vi "ScreenGrabberMain.vi"(8 "Error In":errorcluster, 9 "Grabber Timer":dbl=5.0 min=0.0 max=60.0, 10 "Grab Window every":u32=10 min=10 max=2000 step=10, 11 "Window Title":string="Assetto Corsa") -> (0 "ErrorOut":errorcluster)   [LabVIEW 2018, in "ScreenGrabber.lvlib"]
uses:
  ScreenGrabber.lvlib
  Controls/PreferredControlMethod.ctl
  Controls/PreferredSavingConvention.ctl
  Controls/QueueDriverStates.ctl
  Controls/TemplateDataCluster.ctl
  <vilib>/picture/picture.llb/imagedata.ctl
  System.Drawing
  USER32.DLL
  <vilib>/wsapi/NI_WebServices.lvlib
panel:
  out "Slider":u32(slide) caption="Idle" scale=0.0..100.0
  out "TimerBeforeStart":string
  in  "NamingConvention":T1
  in  "About":bool
  in  "Movement Buttons":T2
  in  "Stop":bool
  in  "Start Grabber":bool
  # "SCREEN GRABBER"
  # "(Verbatim Window Title of  the screen to be grabbed)"
  # "(millisecs)"
  # "(Timer secs)"
  # "Preferred Control"
  # "Naming Convention"
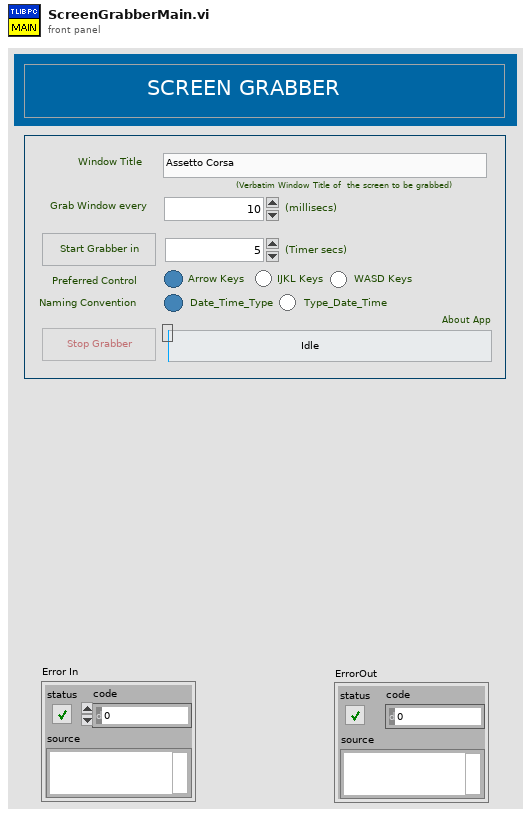
[diagram p1: front panel]
types:
  T1 = typedef "ScreenGrabber.lvlib/PreferredSavingConvention.ctl" = enum32{"Date_Time_Type", "Type_Date_Time"}
  T2 = typedef "ScreenGrabber.lvlib/PreferredControlMethod.ctl" = enum32{"Arrow Keys  ", "IJKL Keys", "WASD Keys"}
  T3 = typedef "ScreenGrabber.lvlib/TemplateDataCluster.ctl" = cluster{"UpVkeyCode":i16, "DownVkeyCode":i16, "LeftVkeyCode":i16, "RightVkeyCode":i16, "WindowHandle":u32, "WindowDimensions":i32[], "WindowWidth":i32, "WindowHeight":i32, "ImageType":u32, "MemoryStreamRef":refnum<k24>, "ImageRef":refnum<k24>, "GraphicsRef":refnum<k24>, "PNGformatRef":refnum<k24>, "ImageSizeRef":refnum<k24>, "CurrentImageData":T4, "SavingConvention":string, "Array of Images":cluster{"CurrentImageData":T4, "Image Path":path}[]}
  T4 = typedef "imagedata.ctl" = cluster{"image type":i32, "image depth":i32, "image":u8[], "mask":u8[], "colors":u32[], "Rectangle":cluster{"left":i16, "top":i16, "right":i16, "bottom":i16}}
  T5 = typedef "ScreenGrabber.lvlib/QueueDriverStates.ctl" = enum16{"Create", "Enqueue", "Enqueue N", "Dequeue", "Enstack", "Enstack N", "Flush", "Destroy"}
  T6 = enum8{"Enabled", "Disabled", "Disabled and Grayed Out"}
  T7 = cluster{"CurrentImageData":T4, "Image Path":path}
  T8 = cluster{"CurrentImageData":T4, "Image Path":path}[]
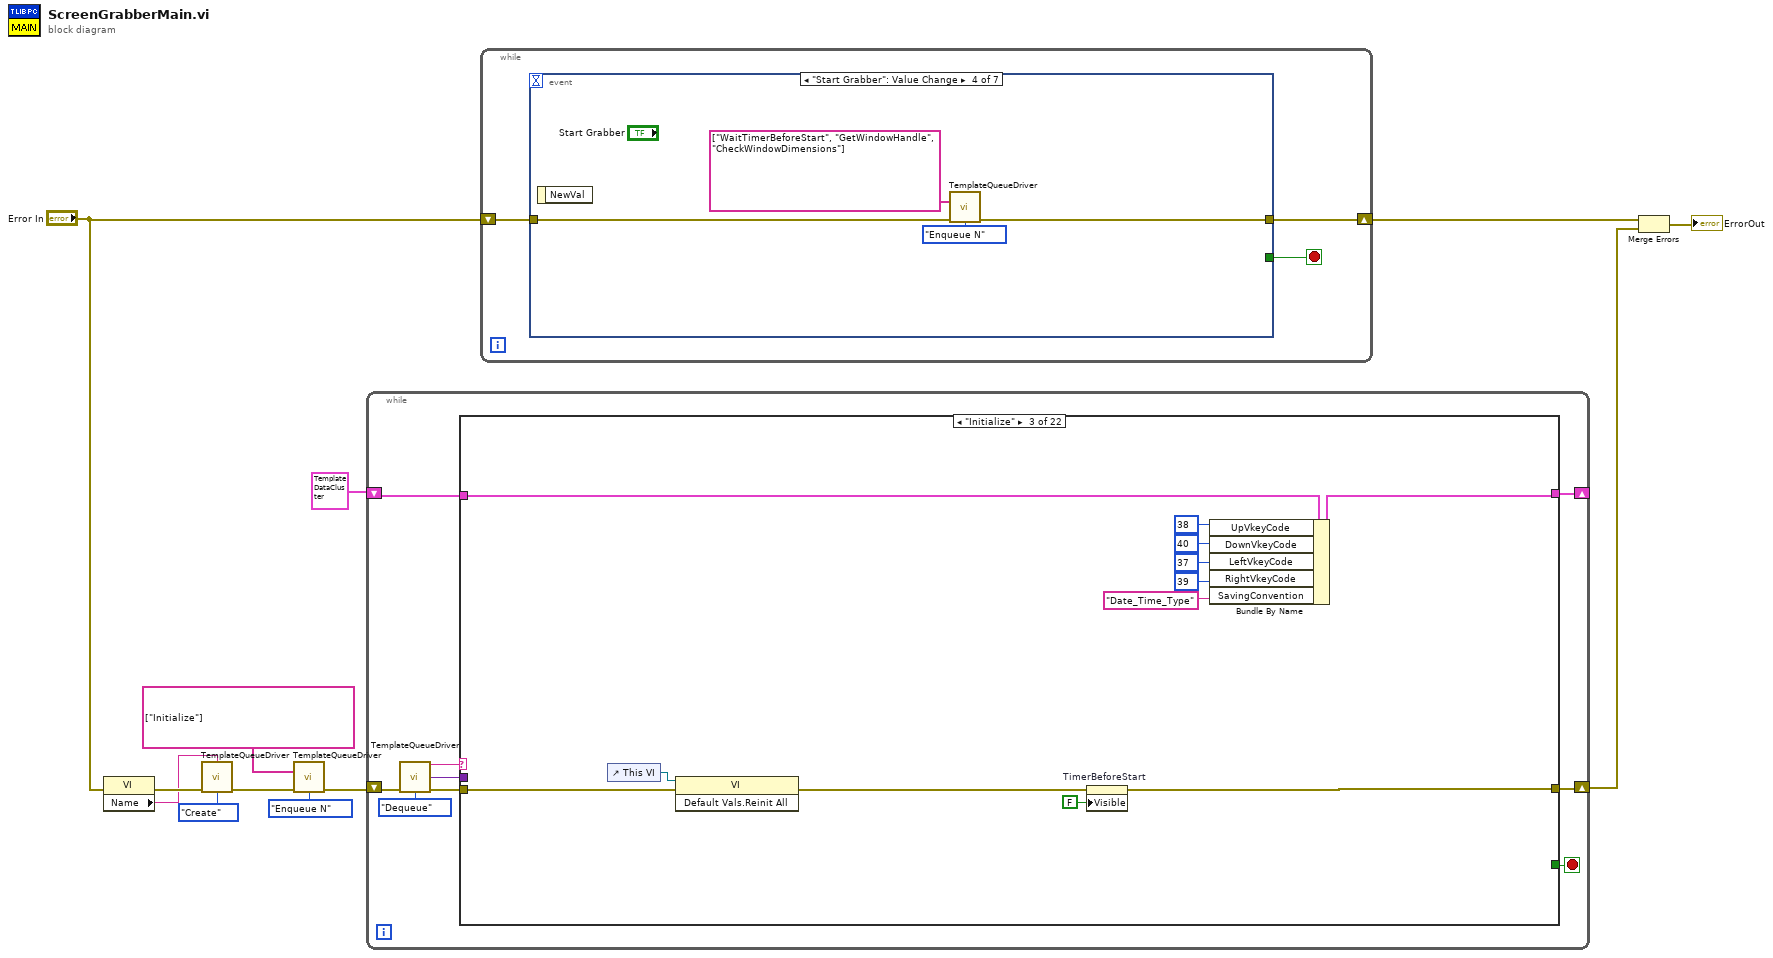
[diagram p0: block diagram]
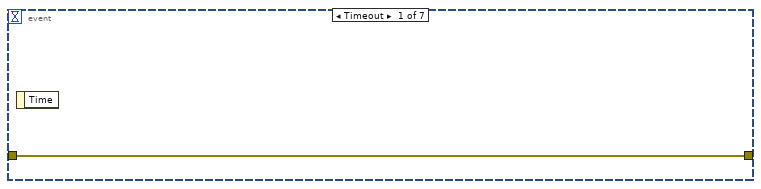
[diagram p2: hidden frame]
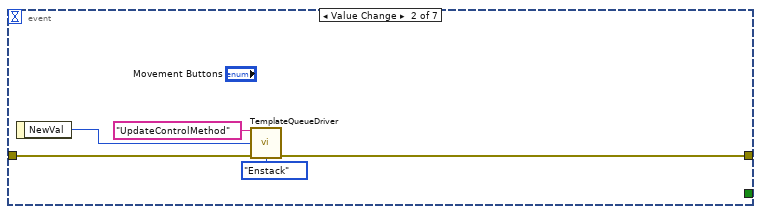
[diagram p3: hidden frame]
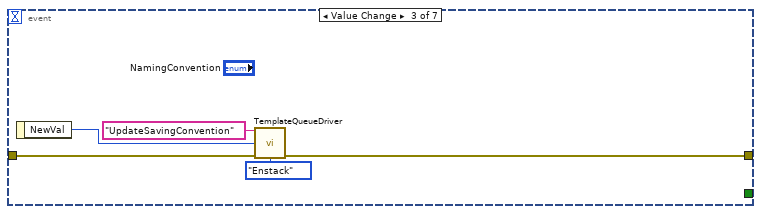
[diagram p4: hidden frame]
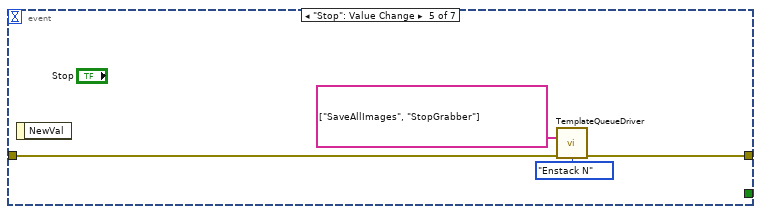
[diagram p5: hidden frame]
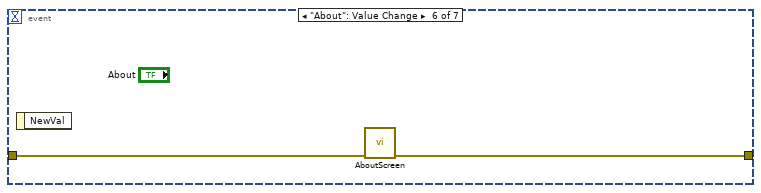
[diagram p6: hidden frame]
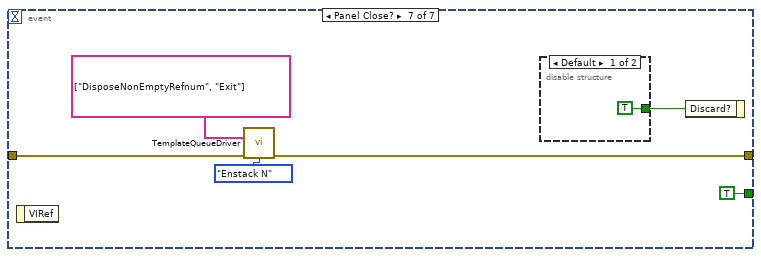
[diagram p7: hidden frame]
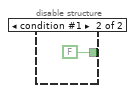
[diagram p8: hidden frame]
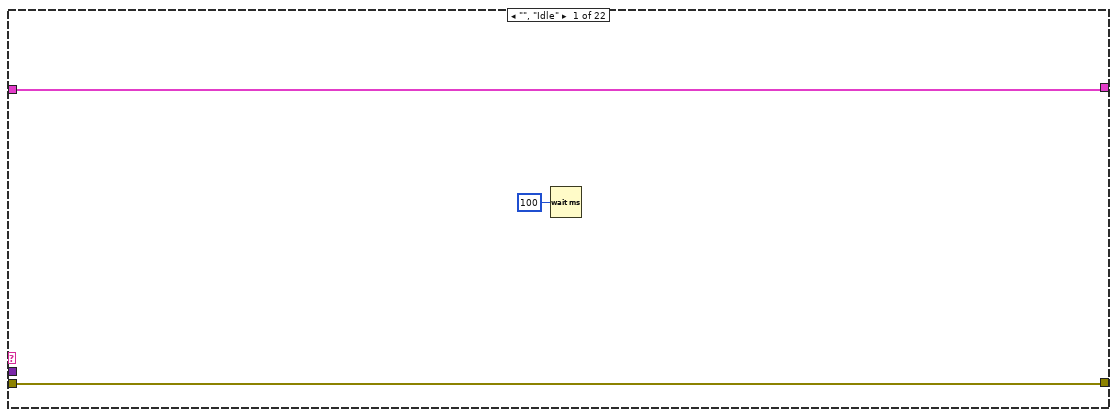
[diagram p9: hidden frame]
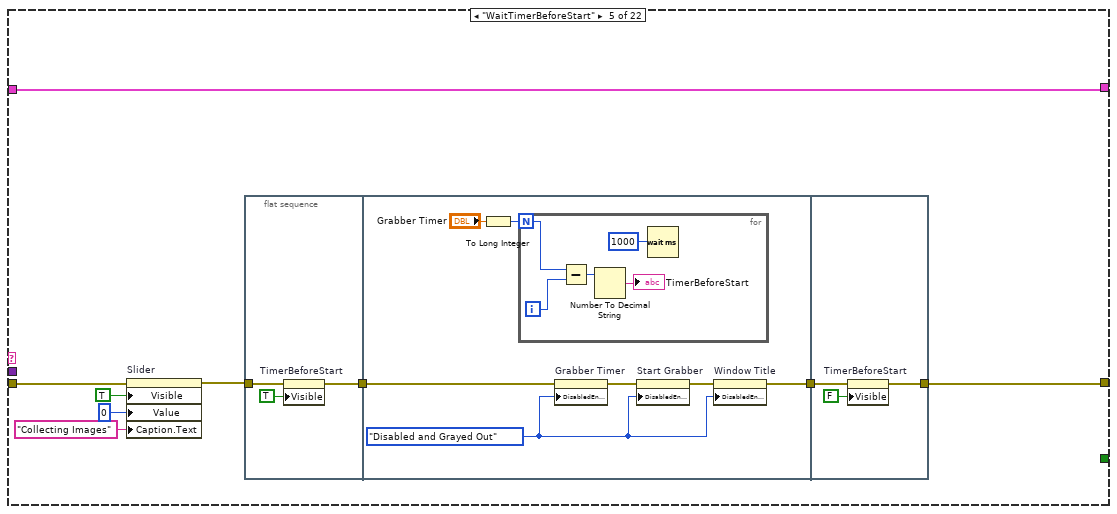
[diagram p12: hidden frame]
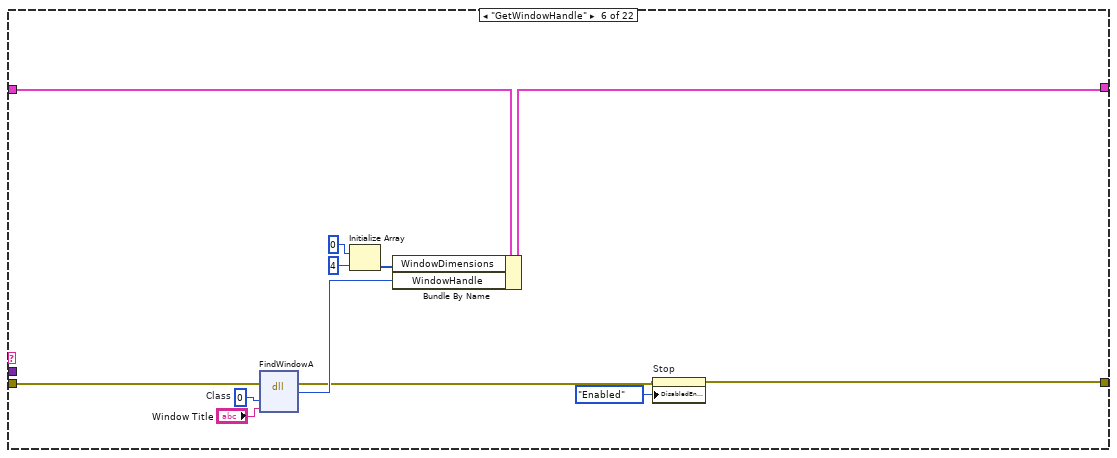
[diagram p13: hidden frame]
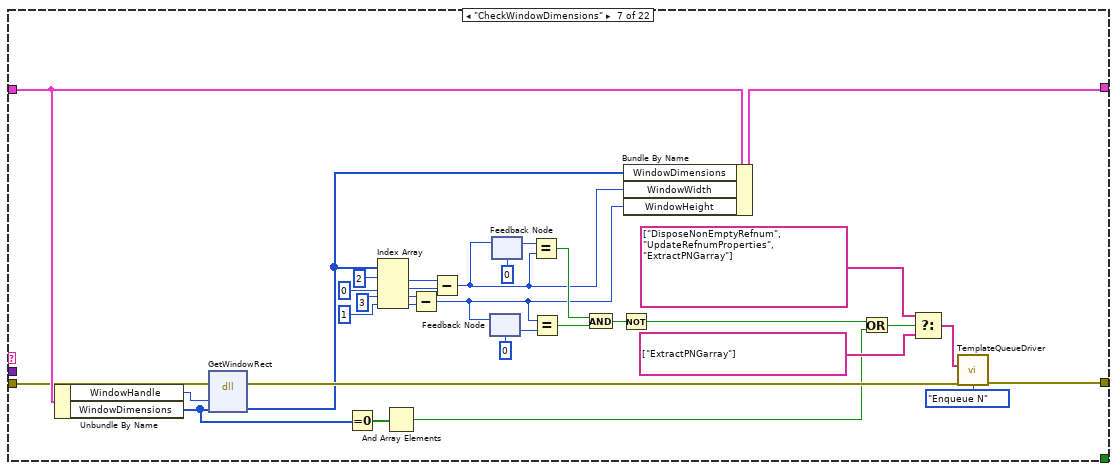
[diagram p14: hidden frame]
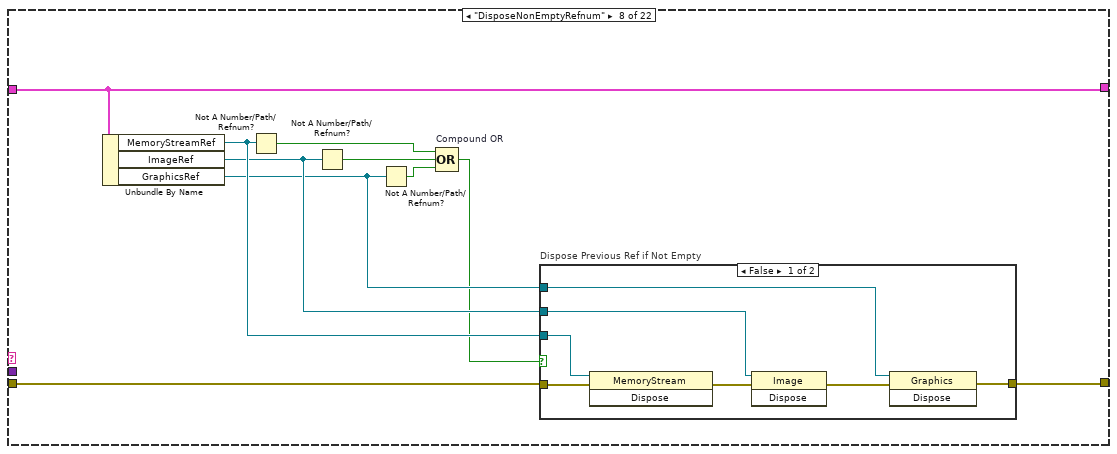
[diagram p15: hidden frame]
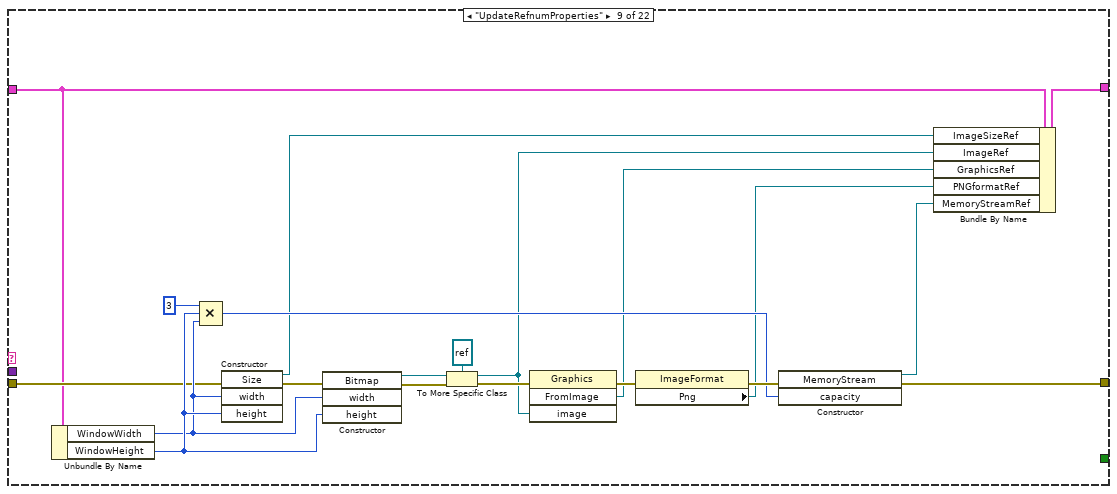
[diagram p17: hidden frame]
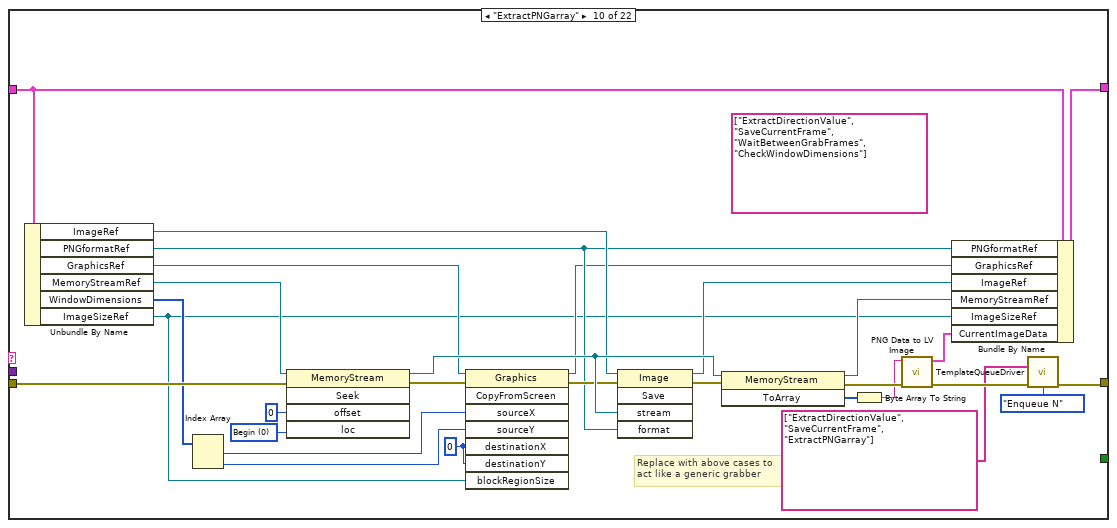
[diagram p18: hidden frame]
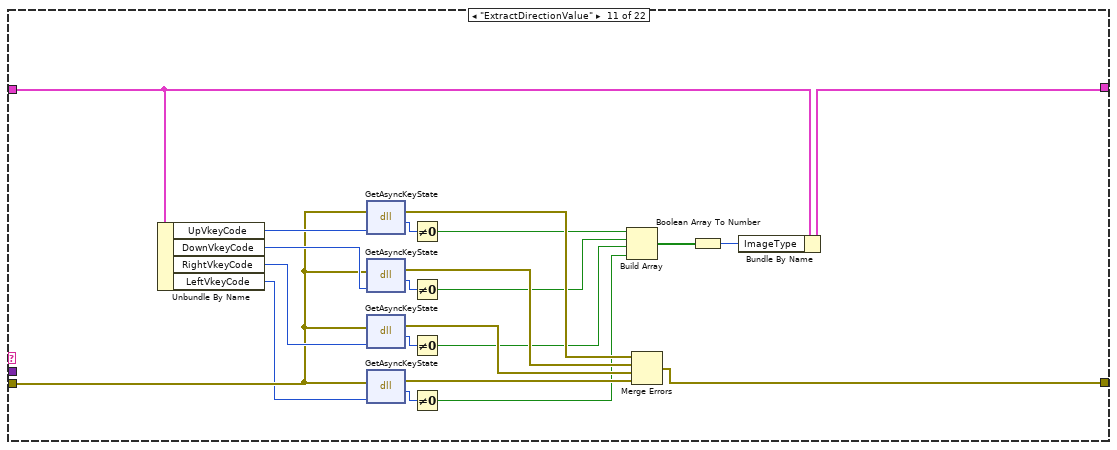
[diagram p19: hidden frame]
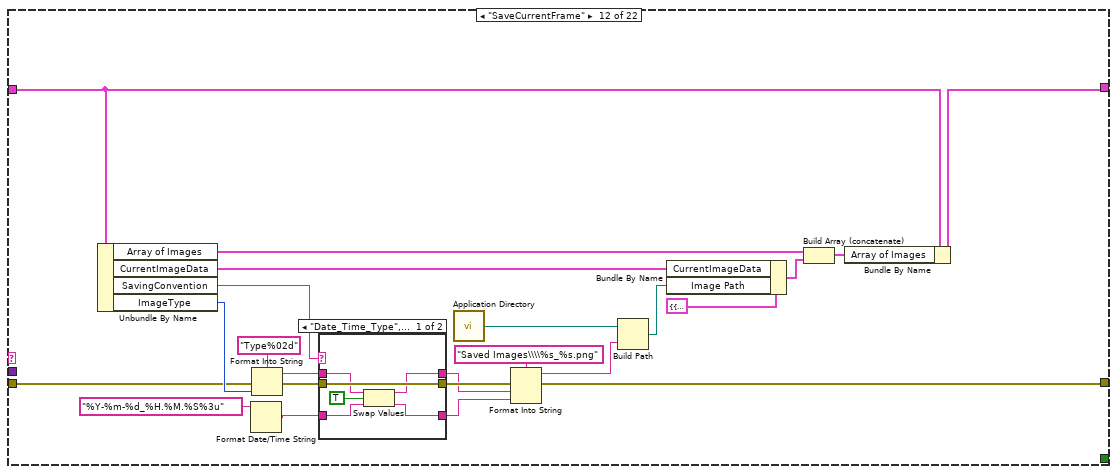
[diagram p20: hidden frame]
diagram:
  n1 = property class="VI"(error in="Error In") -> (error out=w6:errorcluster, "Name"=w5:string)  [unwired: 1 in, 1 out]
  n2 = call "TemplateQueueDriver.vi"("Name"=w5, "ErrorIn"=w6, "Operation"=QueueDriverStates."Create") -> ("ErrorOut"=w12:errorcluster)  [unwired: 10 in, 2 out]
  n3 = call "TemplateQueueDriver.vi"("States[]"=string[] ["Initialize"], "ErrorIn"=w12, "Operation"=QueueDriverStates."Enqueue N") -> ("ErrorOut"=w11:errorcluster)  [unwired: 10 in, 2 out]
  n4 = while {
    shift-right: [w18] -> w10
    shift-left: w11 -> [w21]
    shift-right: [w16] -> _
    shift-left: T3 {"UpVkeyCode"=0, "DownVkeyCode"=0, "LeftVkeyCode"=0, "RightVkeyCode"=0, "WindowHandle"=0, "WindowDimensions"=[], "WindowWidth"=0, "WindowHeight"=0, "ImageType"=0, "MemoryStreamRef"=refnum, "ImageRef"=refnum, "GraphicsRef"=refnum, "PNGformatRef"=refnum, "ImageSizeRef"=refnum, "CurrentImageData"={"image type"=0, "image depth"=0, "image"=[], "mask"=[], "colors"=[], "Rectangle"={"left"=0, "top"=0, "right"=0, "bottom"=0}}, "SavingConvention"="", "Array of Images"=[]} -> [w15]
    stop <- w17 stop-if-true
    n5 = call "TemplateQueueDriver.vi"("ErrorIn"=w21, "Operation"=QueueDriverStates."Dequeue") -> ("State"=w19:string, "Data"=w13:variant, "ErrorOut"=w20:errorcluster)  [unwired: 11 in]
    n6 = case shown="\"Initialize\"" w19 {
      selector: w19 -> [_ _ _ _ _ _ _ _ _ _ _ _ _ _ _ _ _ _ _ _ _ w358]
      tunnel: w20 -> [w24 w26 w36 w40 w45 w79 w110 w121 w138 w171 w189 w204 w236 w249 w285 w299 w310 w331 w333 w336 w342 w357]
      tunnel: [w24 w26 w27 w40 w48 w69 w91 w113 w141 w152 w196 w202 w236 w247 w284 w299 w309 w323 w333 w334 w351 w356] -> w18
      tunnel: [_ _ _ _ _ _ _ _ _ _ _ _ _ _ _ _ _ _ _ _ TRUE _] -> w17
      tunnel: w15 -> [w23 w25 w38 w39 w49 w71 w111 w122 w136 w156 w180 w222 w235 w253 w286 w298 w300 w328 w332 w337 w349 w355]
      tunnel: [w23 w25 w37 w39 w49 w72 w112 w122 w137 w157 w181 w211 w235 w253 w277 w298 w301 w329 w332 w337 w349 w355] -> w16
      tunnel: w13 -> [_ _ _ _ _ _ _ _ _ _ _ _ _ _ _ _ w308 w330 _ _ _ _]
      frame "", "Idle" {
        n7 = Wait (ms)(milliseconds to wait=u32 100) -> ()  [unwired: 1 out]
      }
      frame "---------Initialization---------" {
      }
      frame "Initialize" {
        n8 = control-ref of="This VI"() -> (w35:refnum<vi>)
        n9 = invoke class="VI" method="Default Vals.Reinit All"(reference=w35, error in=w36) -> (error out=w28:errorcluster)  [unwired: 1 in, 2 out]
        n10 = property on="TimerBeforeStart" class="Str"(error in=w28, "Visible"=FALSE) -> (error out=w27:errorcluster)  [unwired: 1 in, 1 out]
        n11 = Bundle By Name(cluster=w38, "UpVkeyCode"=i16 38 ("nvirtkey"), "DownVkeyCode"=i16 40 ("nvirtkey"), "LeftVkeyCode"=i16 37 ("nvirtkey"), "RightVkeyCode"=i16 39 ("nvirtkey"), "SavingConvention"="Date_Time_Type" ("format string")) -> (w37:T3)
      }
      frame "-----------Functions----------" {
      }
      frame "WaitTimerBeforeStart" {
        n12 = property on="Slider" class="Slide (strict)"(error in=w45, "Visible"=TRUE, "Value"=u32 0 ("Slider"), "Caption.Text"="Collecting Images") -> (error out=w44:errorcluster)  [unwired: 1 in, 1 out]
        n13 = flat-sequence {
          tunnel: w44 -> [w51]
          tunnel: [w50] -> w46
          tunnel: [w56] -> w47
          tunnel: w46 -> [w59]
          tunnel: [w65] -> w48
          tunnel: w47 -> [w66]
          frame #0 {
            n14 = property on="TimerBeforeStart" class="Str"(error in=w51, "Visible"=TRUE) -> (error out=w50:errorcluster)  [unwired: 1 in, 1 out]
          }
          frame #1 {
            w55 = T6."Disabled and Grayed Out" ("Disabled")
            n15 = To Long Integer(number="Grabber Timer") -> (32bit integer=w53:i32)
            n16 = for {
              N: w53 -> [w63]
              i -> [w62]
              n17 = Subtract(x=w63, y=w62) -> (x-y=w61:i32)
              n18 = Number To Decimal String(number=w61) -> (decimal integer string=→"TimerBeforeStart":string)  [unwired: 1 in]
              n19 = Wait (ms)(milliseconds to wait=u32 1000 ("y")) -> ()  [unwired: 1 out]
            }
            n20 = property on="Grabber Timer" class="DigNum (strict)"(error in=w59, "DisabledEnum"=w55) -> (error out=w58:errorcluster)  [unwired: 1 in, 1 out]
            n21 = property on="Start Grabber" class="Bool"(error in=w58, "DisabledEnum"=w55) -> (error out=w57:errorcluster)  [unwired: 1 in, 1 out]
            n22 = property on="Window Title" class="Str"(error in=w57, "DisabledEnum"=w55) -> (error out=w56:errorcluster)  [unwired: 1 in, 1 out]
          }
          frame #2 {
            n23 = property on="TimerBeforeStart" class="Str"(error in=w66, "Visible"=FALSE) -> (error out=w65:errorcluster)  [unwired: 1 in, 1 out]
          }
        }
      }
      frame "GetWindowHandle" {
        w77 = 0  # Class
        n24 = dll-call lib="USER32.DLL" fn="FindWindowA"(error in=w79, "class"=w77, "title"="Window Title") -> (error out=w70:errorcluster, "Window Handle"=w76:u32)  [unwired: 4 in, 1 out]
        n25 = Initialize Array(0, 4) -> (w73:i32[])
        n26 = Bundle By Name(cluster=w71, "WindowDimensions"=w73, "WindowHandle"=w76) -> (w72:T3)
        n27 = property on="Stop" class="Bool"(error in=w70, "DisabledEnum"=T6."Enabled" ("Disabled")) -> (error out=w69:errorcluster)  [unwired: 1 in, 1 out]
      }
      frame "CheckWindowDimensions" {
        n28 = Unbundle By Name(w111) -> ("WindowHandle"=w93:u32, "WindowDimensions"=w80:i32[])
        n29 = dll-call lib="USER32.DLL" fn="GetWindowRect"(error in=w110, "hWnd"=w93, "RECT"=w80) -> (error out=w92:errorcluster, "RECT"=w84:i32[])  [unwired: 4 in, 1 out]
        n30 = Equal To 0?(x=w80) -> (x = 0?=w85:bool[])
        n31 = Index Array(array=w84, index #1=2 ("index"), index #2=0 ("index"), index #3=3 ("index"), index #4=1 ("index")) -> (element #1=w105:i32, element #2=w104:i32, element #3=w103:i32, element #4=w102:i32)
        n32 = And Array Elements(Boolean array=w85) -> (logical AND=w81:bool)
        n33 = Subtract(x=w103, y=w102) -> (x-y=w94:i32)
        n34 = Subtract(x=w105, y=w104) -> (x-y=w95:i32)
        n35 = feedback #1(0) -> (w100:i32)
        n36 = feedback-in #1(w94) -> ()
        n37 = feedback #2(0) -> (w101:i32)
        n38 = feedback-in #2(w95) -> ()
        n39 = Equal?(x=w101, y=w95) -> (x = y?=w99:bool)
        n40 = Equal?(x=w94, y=w100) -> (x = y?=w98:bool)
        n41 = And(x=w99, y=w98) -> (x .and. y?=w89:bool)
        n42 = Not(x=w89) -> (.not. x?=w83:bool)
        n43 = Bundle By Name(cluster=w111, "WindowDimensions"=w84, "WindowWidth"=w95, "WindowHeight"=w94) -> (w112:T3)
        n44 = Or(x=w83, y=w81) -> (x .or. y?=w82:bool)
        n45 = Select(t=string[] ["DisposeNonEmptyRefnum", "UpdateRefnumProperties", "ExtractPNGarray"] ("States[]"), s=w82, f=string[] ["ExtractPNGarray"] ("States[]")) -> (s? t:f=w86:string[])
        n46 = call "TemplateQueueDriver.vi"("States[]"=w86, "ErrorIn"=w92, "Operation"=QueueDriverStates."Enqueue N") -> ("ErrorOut"=w91:errorcluster)  [unwired: 10 in, 2 out]
      }
      frame "DisposeNonEmptyRefnum" {
        n47 = Unbundle By Name(w122) -> ("MemoryStreamRef"=w120:refnum<k24>, "ImageRef"=w119:refnum<k24>, "GraphicsRef"=w118:refnum<k24>)
        n48 = Not A Number/Path/Refnum?(number/path/refnum=w120) -> (NaN/Path/Refnum?=w117:bool)
        n49 = Not A Number/Path/Refnum?(number/path/refnum=w119) -> (NaN/Path/Refnum?=w116:bool)
        n50 = Not A Number/Path/Refnum?(number/path/refnum=w118) -> (NaN/Path/Refnum?=w115:bool)
        n51 = Compound Arithmetic op=OR "Compound OR"(w117, w116, w115) -> (w114:bool)
        n52 = case "Dispose Previous Ref if Not Empty" shown="False" w114 {
          tunnel: [w127 w130] -> w113
          tunnel: w121 -> [w126 w130]
          tunnel: w120 -> [w125 _]
          tunnel: w119 -> [w124 _]
          tunnel: w118 -> [w123 _]
          frame False {
            n53 = invoke class="MemoryStream" method="Dispose"(reference=w125, error in=w126) -> (error out=w128:errorcluster)  [unwired: 1 in, 2 out]
            n54 = invoke class="Image" method="Dispose"(reference=w124, error in=w128) -> (error out=w129:errorcluster)  [unwired: 1 in, 2 out]
            n55 = invoke class="Graphics" method="Dispose"(reference=w123, error in=w129) -> (error out=w127:errorcluster)  [unwired: 1 in, 2 out]
          }
          frame True {
          }
        }
      }
      frame "UpdateRefnumProperties" {
        n56 = Unbundle By Name(w136) -> ("WindowWidth"=w139:i32, "WindowHeight"=w144:i32)
        n57 = Compound Arithmetic op=MULTIPLY(3 ("value"), w144, w139) -> (w140:i32)
        n58 = constructor class="Size"(error in=w138, "width"=w139, "height"=w144) -> (reference out=w131:refnum<k24>, error out=w145:errorcluster)  [unwired: 2 in, 3 out]
        n59 = constructor class="Bitmap"(error in=w145, "width"=w139, "height"=w144) -> (reference out=w150:refnum<k24>, error out=w148:errorcluster)  [unwired: 2 in, 3 out]
        n60 = To More Specific Class(target class=refnum<k24> refnum, reference=w150, error in=w148) -> (specific class reference=w132:refnum<k24>, error out=w147:errorcluster)
        n61 = invoke class="Graphics" method="FromImage"(error in=w147, "image"=w132) -> (error out=w146:errorcluster, "FromImage"=w133:refnum<k24>)  [unwired: 2 in, 2 out]
        n62 = property class="ImageFormat"(error in=w146) -> (error out=w142:errorcluster, "Png"=w134:refnum<k24>)  [unwired: 1 in, 1 out]
        n63 = constructor class="MemoryStream"(error in=w142, "capacity"=w140) -> (reference out=w135:refnum<k24>, error out=w141:errorcluster)  [unwired: 2 in, 2 out]
        n64 = Bundle By Name(cluster=w136, "ImageSizeRef"=w131, "ImageRef"=w132, "GraphicsRef"=w133, "PNGformatRef"=w134, "MemoryStreamRef"=w135) -> (w137:T3)
      }
      frame "ExtractPNGarray" {
        (unwired) string[] ["ExtractDirectionValue", "SaveCurrentFrame", "WaitBetweenGrabFrames", "CheckWindowDimensions"] ("States[]")
        w174 = 0 ("destinationX")
        w178 = 0 items=["Begin", "Current", "End"] ("loc")
        # "Replace with above cases to \nact like a generic grabber"
        n65 = Unbundle By Name(w156) -> ("ImageRef"=w165:refnum<k24>, "PNGformatRef"=w163:refnum<k24>, "GraphicsRef"=w166:refnum<k24>, "MemoryStreamRef"=w170:refnum<k24>, "WindowDimensions"=w169:i32[], "ImageSizeRef"=w160:refnum<k24>)
        n66 = Index Array(array=w169) -> (element #1=w167:i32, element #2=w168:i32)  [unwired: 2 in]
        n67 = invoke class="MemoryStream" method="Seek"(reference=w170, error in=w171, "offset"=i64 0, "loc"=w178) -> (reference out=w177:refnum<k24>, error out=w176:errorcluster)  [unwired: 1 in, 3 out]
        n68 = invoke class="Graphics" method="CopyFromScreen"(reference=w166, error in=w176, "sourceX"=w167, "sourceY"=w168, "destinationX"=w174, "destinationY"=w174, "blockRegionSize"=w160) -> (reference out=w161:refnum<k24>, error out=w175:errorcluster)  [unwired: 1 in, 6 out]
        n69 = invoke class="Image" method="Save"(reference=w165, error in=w175, "stream"=w177, "format"=w163) -> (reference out=w162:refnum<k24>, error out=w173:errorcluster)  [unwired: 1 in, 3 out]
        n70 = invoke class="MemoryStream" method="ToArray"(reference=w177, error in=w173) -> (reference out=w164:refnum<k24>, error out=w159:errorcluster, "ToArray"=w172:u8[])  [unwired: 1 in]
        n71 = Byte Array To String(unsigned byte array=w172) -> (string=w158:string)
        n72 = call <vilib>:"PNG Data to LV Image.vi"("error in (no error)"=w159, "png data"=w158) -> ("error out"=w153:errorcluster, "image data"=w155:T4)  [unwired: 8 in]
        n73 = Bundle By Name(cluster=w156, "PNGformatRef"=w163, "GraphicsRef"=w161, "ImageRef"=w162, "MemoryStreamRef"=w164, "ImageSizeRef"=w160, "CurrentImageData"=w155) -> (w157:T3)
        n74 = call "TemplateQueueDriver.vi"("States[]"=string[] ["ExtractDirectionValue", "SaveCurrentFrame", "ExtractPNGarray"], "ErrorIn"=w153, "Operation"=QueueDriverStates."Enqueue N") -> ("ErrorOut"=w152:errorcluster)  [unwired: 10 in, 2 out]
      }
      frame "ExtractDirectionValue" {
        n75 = Unbundle By Name(w180) -> ("UpVkeyCode"=w192:i16, "DownVkeyCode"=w191:i16, "RightVkeyCode"=w190:i16, "LeftVkeyCode"=w188:i16)
        n76 = dll-call lib="user32.dll" fn="GetAsyncKeyState"(error in=w189, "vKey"=w192) -> (error out=w195:errorcluster, "return type"=w198:u16)  [unwired: 3 in, 1 out]
        n77 = dll-call lib="user32.dll" fn="GetAsyncKeyState"(error in=w189, "vKey"=w191) -> (error out=w194:errorcluster, "return type"=w199:u16)  [unwired: 3 in, 1 out]
        n78 = dll-call lib="user32.dll" fn="GetAsyncKeyState"(error in=w189, "vKey"=w190) -> (error out=w193:errorcluster, "return type"=w200:u16)  [unwired: 3 in, 1 out]
        n79 = dll-call lib="user32.dll" fn="GetAsyncKeyState"(error in=w189, "vKey"=w188) -> (error out=w197:errorcluster, "return type"=w201:u16)  [unwired: 3 in, 1 out]
        n80 = Not Equal To 0?(x=w198) -> (x != 0?=w187:bool)
        n81 = Not Equal To 0?(x=w199) -> (x != 0?=w186:bool)
        n82 = Not Equal To 0?(x=w200) -> (x != 0?=w185:bool)
        n83 = Not Equal To 0?(x=w201) -> (x != 0?=w184:bool)
        n84 = Build Array(w187, w186, w185, w184) -> (w183:bool[])
        n85 = Merge Errors(w195, w194, w193, w197) -> (w196:errorcluster)
        n86 = Boolean Array To Number(Boolean array=w183) -> (number=w182:u32)
        n87 = Bundle By Name(cluster=w180, "ImageType"=w182) -> (w181:T3)
      }
      frame "SaveCurrentFrame" {
        n88 = Unbundle By Name(w222) -> ("Array of Images"=w209:T8, "CurrentImageData"=w206:T4, "SavingConvention"=w218:string, "ImageType"=w220:u32)
        n89 = Format Date/Time String(time format string (%c)="%Y-%m-%d_%H.%M.%S%3u") -> (date/time string=w212:string)  [unwired: 2 in]
        n90 = Format Into String(format string="Type%02d", error in=w204, w220) -> (resulting string=w215:string, error out=w217:errorcluster)  [unwired: 1 in]
        n91 = case shown="\"Date_Time_Type\", Default" w218 {
          tunnel: w217 -> [w230 w233]
          tunnel: [w230 w233] -> w216
          tunnel: w215 -> [w229 w232]
          tunnel: w212 -> [w227 w231]
          tunnel: [w228 w232] -> w214
          tunnel: [w226 w231] -> w213
          frame "Date_Time_Type", Default {
            n92 = Swap Values(12:w229, 13:TRUE ("?(T)"), 14:w227) -> (1:w228:string, 3:w226:string)
          }
          frame "Type_Date_Time" {
          }
        }
        n93 = call <vilib>:"Application Directory.vi"() -> ("Application Directory"=w203:path)
        n94 = Format Into String(format string="Saved Images\\\\%s_%s.png", error in=w216, w214, w213) -> (resulting string=w223:string, error out=w202:errorcluster)  [unwired: 1 in]
        n95 = Build Path(base path=w203, name or relative path=w223) -> (appended path=w205:path)
        n96 = Bundle By Name(cluster=T7 {"CurrentImageData"={"image type"=0, "image depth"=0, "image"=[], "mask"=[], "colors"=[], "Rectangle"={"left"=0, "top"=0, "right"=0, "bottom"=0}}, "Image Path"=path ""} ("Cluster"), "CurrentImageData"=w206, "Image Path"=w205) -> (w207:T7)
        n97 = Build Array (concatenate)(w209, w207) -> (w208:T8)
        n98 = Bundle By Name(cluster=w222, "Array of Images"=w208) -> (w211:T3)
      }
      frame "WaitBetweenGrabFrames" {
        n99 = Wait (ms)(milliseconds to wait="Grab Window every") -> ()  [unwired: 1 out]
      }
      frame "SaveAllImages" {
        n100 = call <vilib>:"Set Busy.vi"("error in (no error)"=w249) -> ("error out"=w241:errorcluster)  [unwired: 9 in, 1 out]
        n101 = call <vilib>:"Application Directory.vi"() -> ("Application Directory"=w243:path)
        n102 = Build Path(base path=w243, name or relative path="Saved Images" ("string")) -> (appended path=w244:path)
        n103 = call <vilib>:"Check if File or Folder Exists.vi"("error in (no error)"=w241, "path"=w244) -> ("error out"=w240:errorcluster, "file or folder exists?"=w239:bool, "dup path"=w238:path)  [unwired: 7 in]
        n104 = case "Create Folder\nif necessary" shown="False" w239 {
          tunnel: w240 -> [w256 w257]
          tunnel: [w255 w257] -> w237
          tunnel: w238 -> [w254 _]
          frame False {
            n105 = Create Folder(path (use dialog)=w254, error in=w256) -> (error out=w255:errorcluster)  [unwired: 1 in, 2 out]
          }
          frame True {
          }
        }
        n106 = property on="Stop" class="Bool"(error in=w237, "DisabledEnum"=T6."Disabled and Grayed Out" ("Disabled")) -> (error out=w246:errorcluster)  [unwired: 1 in, 1 out]
        n107 = Unbundle By Name(w253) -> ("Array of Images"=w252:T8)
        n108 = property on="Slider" class="Slide (strict)"(error in=w246, "Visible"=TRUE) -> (error out=w250:errorcluster)  [unwired: 1 in, 1 out]
        n109 = for {
          N -> [w265]
          tunnel: w252 -> [w272] mode=indexing
          tunnel: w250 -> [w273]
          tunnel: [w260] -> w248
          i -> [w266]
          w274 = 1  # Compression
          n110 = Unbundle By Name(w272) -> ("Image Path"=w270:path, "CurrentImageData"=w271:T4)
          n111 = Increment(x=w266) -> (x+1=w264:i32)
          n112 = Divide(x=w264, y=w265) -> (x/y=w269:dbl)
          n113 = Multiply(x=w269, y=100.0) -> (x*y=w267:dbl)
          n114 = call <vilib>:"Write PNG File.vi"("compression (default)"=w274, "error in (no error)"=w273, "image data"=w271, "path to PNG file"=w270) -> ("error out"=w261:errorcluster)  [unwired: 6 in, 1 out]
          n115 = To Unsigned Long Integer(number=w267) -> (unsigned 32bit integer=w259:u32)
          "Slider" <- w259
          n116 = Number To Decimal String(number=w259) -> (decimal integer string=w262:string)  [unwired: 1 in]
          n117 = Concatenate Strings(w262, "% Completed" ("string")) -> (w258:string)
          n118 = property on="Slider" class="Slide (strict)"(error in=w261, "Caption.Text"=w258) -> (error out=w260:errorcluster)  [unwired: 1 in, 1 out]
        }
        n119 = call <vilib>:"Unset Busy.vi"("error in (no error)"=w248) -> ("error out"=w247:errorcluster)  [unwired: 10 in]
      }
      frame "StopGrabber" {
        w282 = T6."Enabled" ("Disabled")
        n120 = property on="Grabber Timer" class="DigNum (strict)"(error in=w285, "DisabledEnum"=w282) -> (error out=w289:errorcluster)  [unwired: 1 in, 1 out]
        n121 = property on="Start Grabber" class="Bool"(error in=w289, "DisabledEnum"=w282) -> (error out=w283:errorcluster)  [unwired: 1 in, 1 out]
        n122 = property on="Window Title" class="Str"(error in=w283, "DisabledEnum"=w282) -> (error out=w275:errorcluster)  [unwired: 1 in, 1 out]
        n123 = Unbundle By Name(w286) -> ("GraphicsRef"=w287:refnum<k24>, "ImageRef"=w288:refnum<k24>, "MemoryStreamRef"=w281:refnum<k24>)
        n124 = call "TemplateQueueDriver.vi"("ErrorIn"=w275, "Operation"=QueueDriverStates."Flush") -> ("ErrorOut"=w278:errorcluster)  [unwired: 11 in, 2 out]
        n125 = Not A Number/Path/Refnum?(number/path/refnum=w281) -> (NaN/Path/Refnum?=w280:bool)
        n126 = case shown="False" w280 {
          tunnel: w288 -> [w294 _]
          tunnel: w287 -> [w293 _]
          tunnel: w278 -> [w292 w297]
          tunnel: [w291 w297] -> w284
          tunnel: w281 -> [w290 _]
          frame False {
            n127 = invoke class="MemoryStream" method="Dispose"(reference=w290, error in=w292) -> (error out=w295:errorcluster)  [unwired: 1 in, 2 out]
            n128 = invoke class="Image" method="Dispose"(reference=w294, error in=w295) -> (error out=w296:errorcluster)  [unwired: 1 in, 2 out]
            n129 = invoke class="Graphics" method="Dispose"(reference=w293, error in=w296) -> (error out=w291:errorcluster)  [unwired: 1 in, 2 out]
          }
          frame True {
          }
        }
        n130 = Bundle By Name(cluster=w286, "Array of Images"=T8 []) -> (w277:T3)
      }
      frame "----------UserEvent-----------" {
      }
      frame "UpdateControlMethod" {
        n131 = Variant To Data(error in=w310, type=PreferredControlMethod."Arrow Keys  " ("Movement Buttons"), Variant=w308) -> (data=w302:T2, error out=w309:errorcluster)
        n132 = case shown="\"WASD Keys\"" w302 {
          tunnel: [i16 38 ("nvirtkey") i16 73 ("nvirtkey") i16 87 ("nvirtkey")] -> w306
          tunnel: [i16 40 ("nvirtkey") i16 75 ("nvirtkey") i16 83 ("nvirtkey")] -> w305
          tunnel: [i16 37 ("nvirtkey") i16 74 ("nvirtkey") i16 65 ("nvirtkey")] -> w304
          tunnel: [i16 39 ("nvirtkey") i16 76 ("nvirtkey") i16 68 ("nvirtkey")] -> w303
          frame "Arrow Keys  ", Default {
          }
          frame "IJKL Keys" {
          }
          frame "WASD Keys" {
          }
        }
        n133 = Bundle By Name(cluster=w300, "UpVkeyCode"=w306, "DownVkeyCode"=w305, "LeftVkeyCode"=w304, "RightVkeyCode"=w303) -> (w301:T3)
      }
      frame "UpdateSavingConvention" {
        n134 = Variant To Data(error in=w331, type=PreferredSavingConvention."Date_Time_Type" ("NamingConvention"), Variant=w330) -> (data=w327:T1, error out=w324:errorcluster)
        n135 = Format Into String(error in=w324, w327) -> (resulting string=w326:string, error out=w323:errorcluster)  [unwired: 2 in]
        n136 = Bundle By Name(cluster=w328, "SavingConvention"=w326) -> (w329:T3)
      }
      frame "--------------Misc------------" {
      }
      frame "Error" {
        # "Case to handle errors"
        n137 = call <vilib>:"Simple Error Handler.vi"("error in (no error)"=w336) -> ("error out"=w335:errorcluster)  [unwired: 4 in, 4 out]
        n138 = call <vilib>:"Clear Errors.vi"("error in (no error)"=w335) -> ("error out"=w334:errorcluster)  [unwired: 5 in, 1 out]
      }
      frame "Exit" {
        w346 = T6."Enabled" ("Disabled")
        # "Case to exit the VI"
        n139 = property on="Slider" class="Slide (strict)"(error in=w342, "Visible"=TRUE, "Value"=u32 0 ("Slider"), "Caption.Text"="Idle") -> (error out=w341:errorcluster)  [unwired: 1 in, 1 out]
        n140 = property on="Grabber Timer" class="DigNum (strict)"(error in=w341, "DisabledEnum"=w346) -> (error out=w348:errorcluster)  [unwired: 1 in, 1 out]
        n141 = property on="Start Grabber" class="Bool"(error in=w348, "DisabledEnum"=w346) -> (error out=w347:errorcluster)  [unwired: 1 in, 1 out]
        n142 = property on="Window Title" class="Str"(error in=w347, "DisabledEnum"=w346) -> (error out=w340:errorcluster)  [unwired: 1 in, 1 out]
        n143 = property on="Stop" class="Bool"(error in=w340, "DisabledEnum"=T6."Disabled and Grayed Out" ("Disabled")) -> (error out=w339:errorcluster)  [unwired: 1 in, 1 out]
        n144 = call "TemplateQueueDriver.vi"("ErrorIn"=w339, "Operation"=QueueDriverStates."Destroy") -> ("ErrorOut"=w351:errorcluster)  [unwired: 11 in, 2 out]
      }
      frame "False", Default {
        # "Case to handle undefined case stirngs"
        n145 = Concatenate Strings("No case for this string \"" ("string"), w358, "\" in ScreenGrabber Main module" ("string")) -> (w360:string)
        n146 = One Button Dialog(message=w360, button name ("OK")="OK") -> ()  [unwired: 1 out]
        n147 = call "TemplateQueueDriver.vi"("State"="Exit", "ErrorIn"=w357, "Operation"=QueueDriverStates."Enqueue") -> ("ErrorOut"=w356:errorcluster)  [unwired: 10 in, 2 out]
      }
    }
  }
  n148 = while {
    shift-right: [w363] -> w7
    shift-left: "Error In" -> [w365]
    stop <- w364 stop-if-true
    n149 = event shown="[3] \"Start Grabber\": Value Change" {
      selector: _ -> [_ _ _ _ _ _ _]
      dyn-events: _ -> [_ _ _ _ _ _ _]
      timeout: _ -> [_ _ _ _ _ _ _]
      tunnel: w365 -> [w366 w371 w376 w379 w383 w386 w392]
      tunnel: [w366 w370 w375 w377 w381 w385 w391] -> w363
      tunnel: [_ _ _ _ _ _ TRUE] -> w364
      event Timeout {
        n150 = event-data() -> ()  [unwired: 1 in, 1 out]
      }
      event Value Change {
        n151 = event-data() -> ("NewVal"=w368:T2)  [unwired: 1 in]
        n152 = call "TemplateQueueDriver.vi"("State"="UpdateControlMethod", "Data"=w368, "ErrorIn"=w371, "Operation"=QueueDriverStates."Enstack") -> ("ErrorOut"=w370:errorcluster)  [unwired: 9 in, 2 out]
      }
      event Value Change {
        n153 = event-data() -> ("NewVal"=w373:T1)  [unwired: 1 in]
        n154 = call "TemplateQueueDriver.vi"("State"="UpdateSavingConvention", "Data"=w373, "ErrorIn"=w376, "Operation"=QueueDriverStates."Enstack") -> ("ErrorOut"=w375:errorcluster)  [unwired: 9 in, 2 out]
      }
      event "Start Grabber": Value Change {
        n155 = event-data() -> ()  [unwired: 1 in, 1 out]
        n156 = call "TemplateQueueDriver.vi"("States[]"=string[] ["WaitTimerBeforeStart", "GetWindowHandle", "CheckWindowDimensions"], "ErrorIn"=w379, "Operation"=QueueDriverStates."Enqueue N") -> ("ErrorOut"=w377:errorcluster)  [unwired: 10 in, 2 out]
      }
      event "Stop": Value Change {
        n157 = event-data() -> ()  [unwired: 1 in, 1 out]
        n158 = call "TemplateQueueDriver.vi"("States[]"=string[] ["SaveAllImages", "StopGrabber"], "ErrorIn"=w383, "Operation"=QueueDriverStates."Enstack N") -> ("ErrorOut"=w381:errorcluster)  [unwired: 10 in, 2 out]
      }
      event "About": Value Change {
        n159 = event-data() -> ()  [unwired: 1 in, 1 out]
        n160 = call "AboutScreen.vi"("error in (no error)"=w386) -> ("error out"=w385:errorcluster)  [unwired: 10 in]
      }
      event Panel Close? {
        n161 = event-data() -> ()  [unwired: 1 in, 1 out]
        n162 = call "TemplateQueueDriver.vi"("States[]"=string[] ["DisposeNonEmptyRefnum", "Exit"], "ErrorIn"=w392, "Operation"=QueueDriverStates."Enstack N") -> ("ErrorOut"=w391:errorcluster)  [unwired: 10 in, 2 out]
        n163 = disable-structure shown="Default" {
          disable-tunnel: [TRUE FALSE] -> w390
          frame condition #0 (active) {
          }
          frame condition #1 {
          }
        }
        n164 = event-data("Discard?"=w390) -> ()  [unwired: 1 in, 1 out]
      }
    }
  }
  n165 = Merge Errors(w7, w10) -> (→"ErrorOut":errorcluster)
